vi "knob global.vi"() -> ()   [LabVIEW 2016]
panel:
  in  "Knob type":string="Phidgets 3-axis USB knob box"
  in  "Encoder resolution (1/turn)":dbl=80.0
  in  "Serial numbers":i32[](array[numeric])=[82336, 82363, 82376]
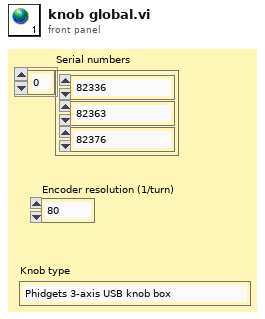
[diagram p1: front panel]
diagram:
